vi "PhyicalChannelConvertor_V0.vi"(10 "Device Name":tag, 11 "Channel Number Array":i32[](array[numeric])) -> (2 "physical channels":tag)   [LabVIEW 2021]
doc: "This vi helps to covert an array of Channel Number and Device name into actual physical channels."
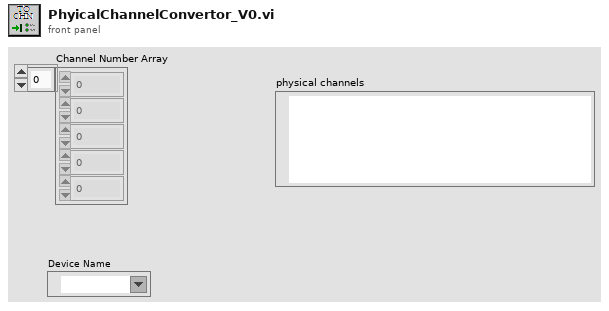
[diagram p1: front panel]
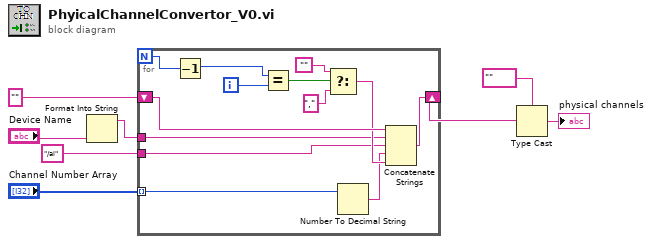
[diagram p0: block diagram]
diagram:
  n1 = Format Into String("Device Name") -> (resulting string=w1:string)  [unwired: 3 in, 1 out]
  n2 = for {
    N -> [w15]
    tunnel: "Channel Number Array" -> [w9] mode=indexing
    shift-right: [w21] -> w3
    shift-left: "" -> [w20]
    tunnel: "/ai" ("string") -> [w10]
    tunnel: w1 -> [w11]
    i -> [w17]
    n3 = Decrement(x=w15) -> (x-1=w14:i32)
    n4 = Equal?(x=w14, y=w17) -> (x = y?=w16:bool)
    n5 = Select(t="", s=w16, f="," ("string")) -> (s? t:f=w13:string)
    n6 = Number To Decimal String(number=w9) -> (decimal integer string=w12:string)  [unwired: 1 in]
    n7 = Concatenate Strings(w20, w11, w10, w12, w13) -> (w21:string)
  }
  n8 = Type Cast(type=tag "" ("physical channels"), x=w3) -> (*(type *) &x=→"physical channels":tag)
